vi "FRIC_navX_Get_LinearAcceleration.vi"(6 "Zero":bool, 7 "Update":bool) -> (2 "Linear Acceleration":T1)   [LabVIEW 2015, in "navX AE v1.lvlib"]
doc: "This navX VI returns the linear acceleration from the navX."
uses:
  navX AE v1.lvlib
  navX Library v2/_TypeDefs/Z900_navX_DeviceRegisters.ctl
  navX Library v2/navX Library v2.lvlib
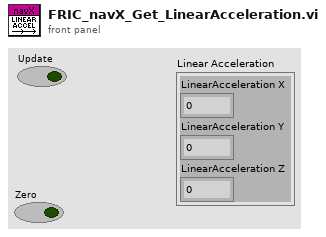
[diagram p1: front panel]
types:
  T1 = cluster{"LinearAcceleration X":dbl, "LinearAcceleration Y":dbl, "LinearAcceleration Z":dbl}
  T2 = typedef "navX Library v2.lvlib/Z900_navX_DeviceRegisters.ctl" = u8
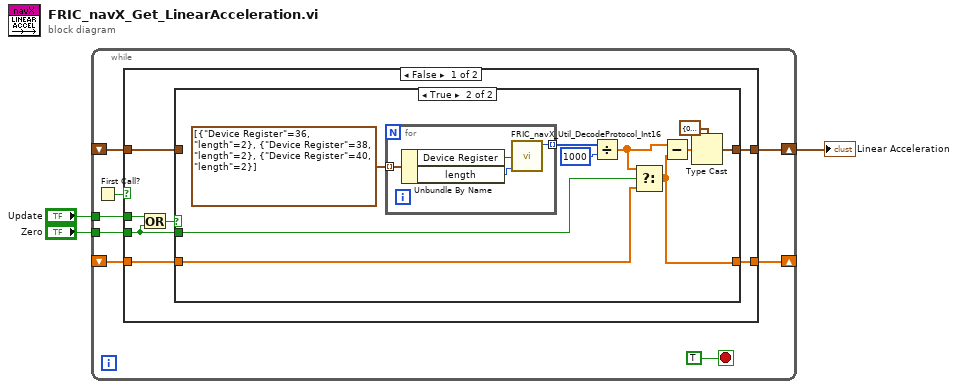
[diagram p0: block diagram]
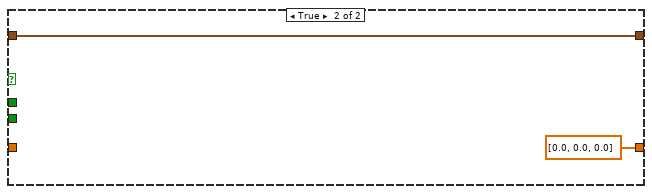
[diagram p3: hidden frame]
diagram:
  n1 = while {
    shift-right: [w11] -> w3
    shift-left: _ -> [w8]
    tunnel: "Update" -> [w9]
    tunnel: "Zero" -> [w6]
    shift-right: [w4] -> _
    shift-left: _ -> [w5]
    stop <- TRUE stop-if-true
    n2 = First Call?() -> (First Call?: T/F=w7:bool)
    n3 = case shown="False" w7 {
      tunnel: [w18 w35] -> w11
      tunnel: w9 -> [w16 _]
      tunnel: w8 -> [w17 w35]
      tunnel: w6 -> [w14 _]
      tunnel: w5 -> [w13 _]
      tunnel: [w12 dbl[] [0.0, 0.0, 0.0]] -> w4
      frame False {
        n4 = Or(x=w16, y=w14) -> (x .or. y?=w15:bool)
        n5 = case shown="True" w15 {
          tunnel: [w20 w30] -> w18
          tunnel: w17 -> [w20 _]
          tunnel: w14 -> [_ w23]
          tunnel: w13 -> [w19 w22]
          tunnel: [w19 w21] -> w12
          frame False {
          }
          frame True {
            n6 = for {
              tunnel: cluster{"Device Register":T2, "length":i32}[] [{"Device Register"=36, "length"=2}, {"Device Register"=38, "length"=2}, {"Device Register"=40, "length"=2}] ("Array") -> [w32] mode=indexing
              tunnel: [w31] -> w26 mode=indexing
              n7 = Unbundle By Name(w32) -> ("Device Register"=w34:T2, "length"=w33:i32)
              n8 = call "FRIC_navX_Util_DecodeProtocol_Int16.vi"("length"=w33, "Device Register"=w34) -> ("Value"=w31:i16)  [unwired: 9 in]
            }
            n9 = Divide(x=w26, y=1000) -> (x/y=w24:dbl[])
            n10 = Select(t=w24, s=w23, f=w22) -> (s? t:f=w21:dbl[])
            n11 = Subtract(x=w24, y=w21) -> (x-y=w25:dbl[])
            n12 = Type Cast(type=T1 {"LinearAcceleration X"=0.0, "LinearAcceleration Y"=0.0, "LinearAcceleration Z"=0.0}, x=w25) -> (*(type *) &x=w30:T1)
          }
        }
      }
      frame True {
      }
    }
  }
  "Linear Acceleration" <- w3
